vi "Get Child Hwnd[].vi"(0 "Doc Class Object[]":refnum<class "Document.lvclass">[](array[class]), 11 "error in (no error)":errorcluster) -> (4 "Doc Class Object[]  2":refnum<class "Document.lvclass">[](array[class]), 6 "ChildHwnd[]":u32[](array[numeric]), 15 "error out":errorcluster)   [LabVIEW 2016, in "Document.lvclass"]
uses:
  Document.lvclass
  Document.lvclass/Document.ctl
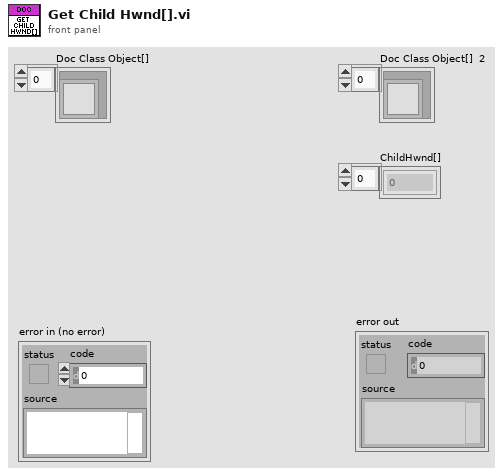
[diagram p1: front panel]
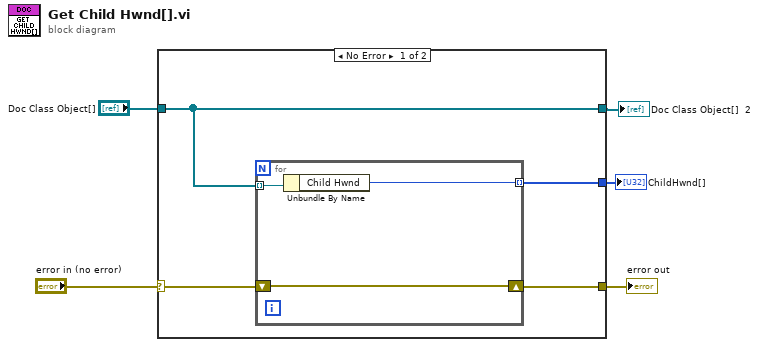
[diagram p0: block diagram]
diagram:
  n1 = case shown="No Error" "error in (no error)" {
    selector: "error in (no error)" -> [w9 w14]
    tunnel: [w8 w14] -> w4
    tunnel: [w7 w13] -> w1
    tunnel: "Doc Class Object[]" -> [w7 w13]
    tunnel: [w6 _] -> w3
    frame No Error {
      n2 = for {
        shift-right: [w12] -> w8
        shift-left: w9 -> [w12]
        tunnel: [w10] -> w6 mode=indexing
        tunnel: w7 -> [w11] mode=indexing
        n3 = Unbundle By Name(w11) -> ("Child Hwnd"=w10:u32)
      }
    }
    frame Error {
    }
  }
  "error out" <- w4
  "ChildHwnd[]" <- w3
  "Doc Class Object[]  2" <- w1
